vi "SendAudioData.vi"(8 "error in (no error)":errorcluster, 10 "Audio":waveform(dbl)) -> (0 "error out":errorcluster)   [LabVIEW 2019, in "Audio Input.lvlib"]
doc: "This event broadcasts captured audio waveform \n_____\nCreated using Delacor QMH Event Scripter 4.2.1.88."
uses:
  Audio Input.lvlib
  SendAudioData Argument--cluster.ctl
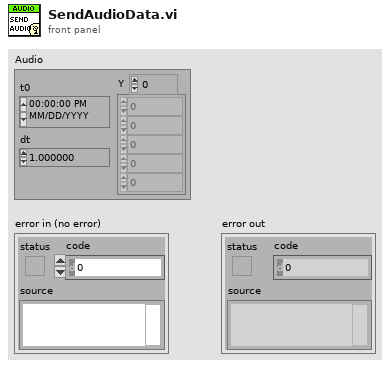
[diagram p1: front panel]
types:
  T1 = typedef "Audio Input.lvlib/SendAudioData Argument--cluster.ctl" = cluster{"Audio":waveform(dbl)}
  T2 = typedef "Audio Input.lvlib/Broadcast Events--cluster.ctl" = cluster{"Module Did Init":refnum<user-event>, "Status Updated":refnum<user-event>, "Error Reported":refnum<user-event>, "Module Did Stop":refnum<user-event>, "Update Module Execution Status":refnum<user-event>, "SendAudioData":refnum<user-event>}
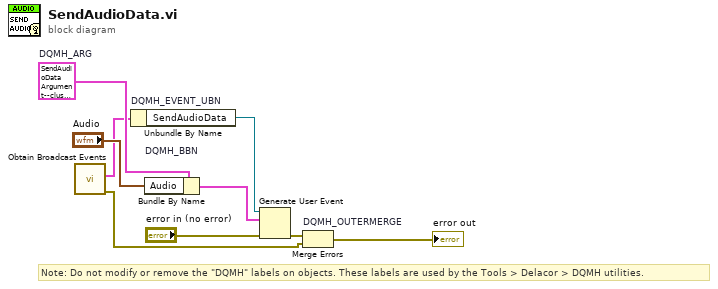
[diagram p0: block diagram]
diagram:
  w4 = T1 {"Audio"={"t0"=timestamp(0 s since 1904-01-01), "dt"=1.0, "Y"=[]}}  # DQMH_ARG
  # "Note: Do not modify or remove the \"DQMH\" labels on objects. These labels are used by the Tools > Delacor > DQMH utilities."
  n1 = call "Obtain Broadcast Events.vi"() -> ("error out"=w2:errorcluster, "Audio Input Broadcast Events"=w1:T2)  [unwired: 10 in]
  n2 = Unbundle By Name "DQMH_EVENT_UBN"(w1) -> ("SendAudioData"=w6:refnum<user-event>)
  n3 = Bundle By Name "DQMH_BBN"(cluster=w4, "Audio"="Audio") -> (w7:T1)
  n4 = Generate User Event(user event=w6, event data cluster=w7, error in="error in (no error)") -> (error out=w5:errorcluster)  [unwired: 1 in, 1 out]
  n5 = Merge Errors "DQMH_OUTERMERGE"(w5, w2) -> (→"error out":errorcluster)
